vi "tokenize_string.vi"(8 "error in (no error)":errorcluster, 10 "delimiter":string, 11 "input_string":string) -> (0 "error out":errorcluster, 3 "delimited_string []":string[](array[string]))   [LabVIEW 2015, in "lv-pagination.lvlib"]
uses:
  lv-pagination.lvlib
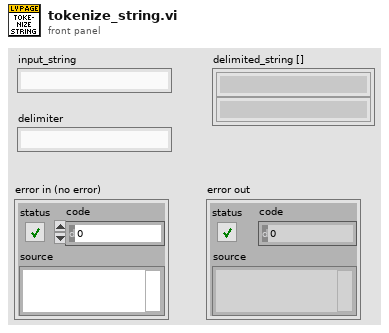
[diagram p1: front panel]
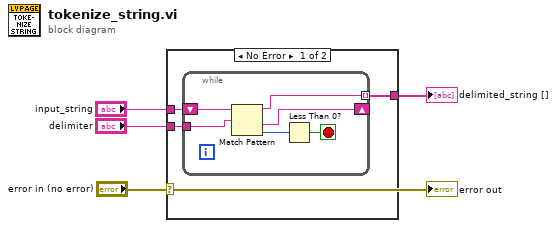
[diagram p0: block diagram]
diagram:
  n1 = case shown="No Error" "error in (no error)" {
    tunnel: "delimiter" -> [w7 _]
    tunnel: [w6 _] -> w3
    tunnel: "input_string" -> [w5 _]
    frame No Error {
      n2 = while {
        shift-right: [w11] -> _
        shift-left: w5 -> [w13]
        tunnel: [w12] -> w6 mode=indexing
        tunnel: w7 -> [w8]
        stop <- w9 stop-if-true
        n3 = Match Pattern(string=w13, regular expression=w8) -> (before substring=w12:string, after substring=w11:string, offset past match=w10:i32)  [unwired: 1 in, 1 out]
        n4 = Less Than 0?(x=w10) -> (x < 0?=w9:bool)
      }
    }
    frame Error {
    }
  }
  "delimited_string []" <- w3
  "error out" <- "error in (no error)"
